vi "Write Lines.vi"(8 "error in (no error)":errorcluster, 10 "Lines":T1[](array[typedef]), 11 "Add Module configuration in":refnum<class "Add Module configuration.lvclass">) -> (0 "error out":errorcluster, 3 "Add Module configuration out":refnum<class "Add Module configuration.lvclass">)   [LabVIEW 2018, in "Add Module configuration.lvclass"]
uses:
  Add Module configuration.lvclass
  Line.ctl
  <vilib>/NI/Tag Bus Module Framework/channel/TBM channel.lvclass
  Add Module configuration.lvclass/Add Module configuration.ctl
  <vilib>/NI/Tag Bus Module Framework/module configuration/TBM module configuration.lvclass
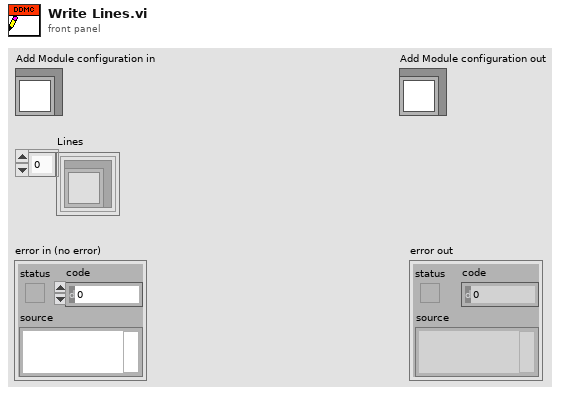
[diagram p1: front panel]
types:
  T1 = typedef "Add Module configuration.lvclass/Line.ctl" = cluster{"channel":refnum<class "TBM channel.lvclass">}
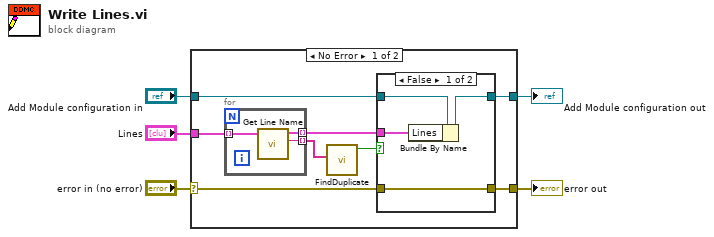
[diagram p0: block diagram]
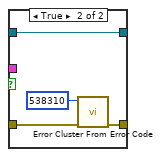
[diagram p2: hidden frame]
diagram:
  n1 = case shown="No Error" "error in (no error)" {
    selector: "error in (no error)" -> [w11 w25]
    tunnel: [w10 w25] -> w4
    tunnel: [w6 w26] -> w2
    tunnel: "Add Module configuration in" -> [w7 w26]
    tunnel: "Lines" -> [w13 _]
    frame No Error {
      n2 = for {
        tunnel: w13 -> [w24] mode=indexing
        tunnel: [w23] -> w12 mode=indexing
        tunnel: [w22] -> w8 mode=indexing
        n3 = call "Get Line Name.vi"("Line in"=w24) -> ("Name"=w23:string, "Line out"=w22:T1)  [unwired: 8 in, 1 out]
      }
      n4 = call <vilib>:"FindDuplicate.vi"("Array"=w12) -> ("Duplicate"=w9:bool)  [unwired: 8 in, 2 out]
      n5 = case shown="False" w9 {
        tunnel: w11 -> [w17 w20]
        tunnel: [w17 w19] -> w10
        tunnel: w8 -> [w15 _]
        tunnel: w7 -> [w16 w18]
        tunnel: [w14 w18] -> w6
        frame False {
          n6 = Bundle By Name(cluster=w16, "Lines"=w15) -> (w14:refnum<class "Add Module configuration.lvclass">)
        }
        frame True {
          n7 = call <vilib>:"Error Cluster From Error Code.vi"("error in (no error)"=w20, "error code (0)"=538310) -> ("error out"=w19:errorcluster)  [unwired: 7 in]
        }
      }
    }
    frame Error {
    }
  }
  "error out" <- w4
  "Add Module configuration out" <- w2
